vi "Chart[Template].TestLauncher.vi"() -> ()   [LabVIEW 2013, in "Chart[Template].lvclass"]
doc: "JKI State Machine Objects (SMO) 1.0.0.5\nJKI - JKI\nCopyright (c) 2016, JKI"
uses:
  Chart[Template].lvclass
  Typedefs/Dependencies--Cluster.ctl
  <vilib>/JKI/JKI SMO/SMO/SMO.lvclass
  <vilib>/JKI/JKI SMO/SMO.UI/SMO.UI.lvclass
panel:
  in  "Send":bool
  out "error out":errorcluster
  in  "Stop":bool
  # "Chart Test Launcher"
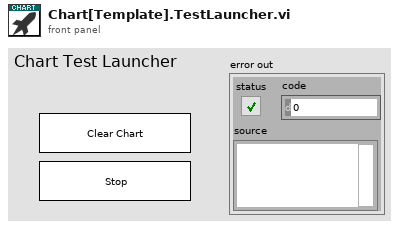
[diagram p1: front panel]
types:
  T1 = typedef "Chart[Template].lvclass/Dependencies--Cluster.ctl" = cluster{"SMO":refnum<class "SMO.lvclass">, "New Value":refnum<user-event>}
  T2 = cluster{"Chart[Template] Public Events":refnum<event-registration>, "SMO.UI Public Events":refnum<event-registration>}
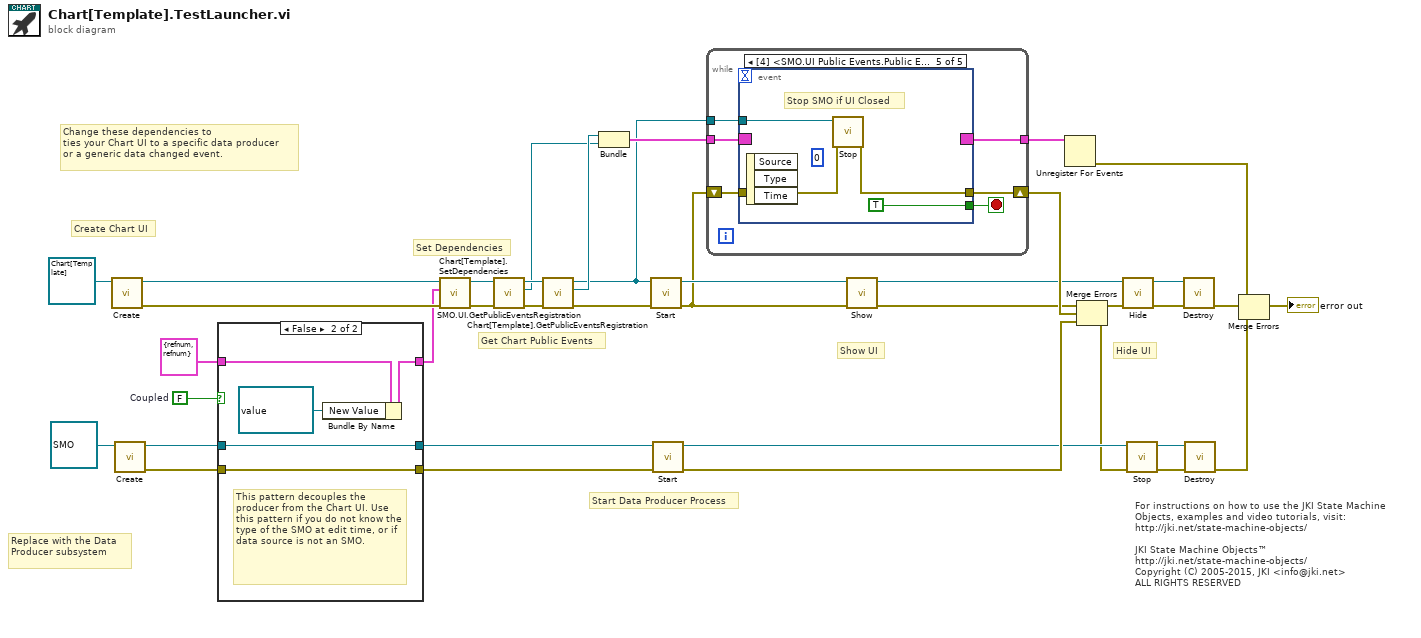
[diagram p0: block diagram]
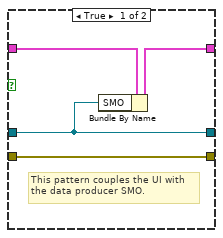
[diagram p2: hidden frame]
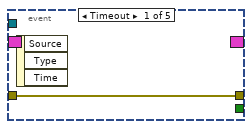
[diagram p3: hidden frame]
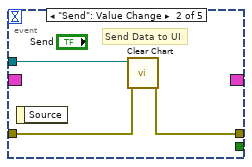
[diagram p4: hidden frame]
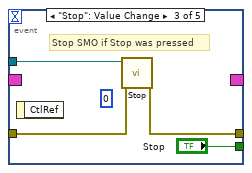
[diagram p5: hidden frame]
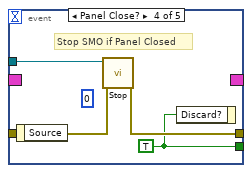
[diagram p6: hidden frame]
diagram:
  w5 = FALSE  # Coupled
  # "Start Data Producer Process"
  # "Set Dependencies"
  # "Create Chart UI"
  # "Replace with the Data Producer subsystem"
  # "Change these dependencies to\nties your Chart UI to a specific data producer\nor a generic data changed event."
  # "Hide UI"
  # "Show UI"
  # "For instructions on how to use the JKI State Machine Objects, examples and video tutorials, visit:\nhttp://jki.net/state-machine-objects/\n\nJKI State Machine Objects™\nhttp://jki.net/state-machine-objects/\nCopyright (C) 2005-2015, JKI <info@jki.net>\nALL RIGHTS RESERVED"
  # "Get Chart Public Events"
  n1 = call <vilib>:"Create.vi"("SMO"=refnum<class "Chart[Template].lvclass"> refnum ("Chart[Template]")) -> ("error out"=w16:errorcluster, "SMO out"=w18:refnum<class "Chart[Template].lvclass">)  [unwired: 8 in, 1 out]
  n2 = call <vilib>:"Create.vi"("SMO"=refnum<class "SMO.lvclass"> refnum) -> ("error out"=w1:errorcluster, "SMO out"=w4:refnum<class "SMO.lvclass">)  [unwired: 8 in, 1 out]
  n3 = case shown="False" w5 {
    tunnel: T1 {"SMO"=refnum, "New Value"=refnum} ("Dependencies") -> [w41 w46]
    tunnel: [w40 w45] -> w6
    tunnel: w4 -> [w39 w43]
    tunnel: [w39 w43] -> w3
    tunnel: [w38 w42] -> w2
    tunnel: w1 -> [w38 w42]
    frame True {
      # "This pattern couples the UI with\nthe data producer SMO."
      n4 = Bundle By Name(cluster=w41, "SMO"=w39) -> (w40:T1)
    }
    frame False {
      # "This pattern decouples the producer from the Chart UI. Use this pattern if you do not know the type of the SMO at edit time, or if data source is not an SMO."
      n5 = Bundle By Name(cluster=w46, "New Value"=refnum<user-event> refnum) -> (w45:T1)
    }
  }
  n6 = call "Chart[Template].SetDependencies.vi"("error in (no error)"=w16, "Dependencies"=w6, "Chart[Template]"=w18) -> ("error out"=w15:errorcluster, "Chart[Template] out"=w17:refnum<class "Chart[Template].lvclass">)  [unwired: 7 in]
  n7 = call <vilib>:"SMO.UI.GetPublicEventsRegistration.vi"("error in (no error)"=w15, "SMO.UI"=w17) -> ("error out"=w21:errorcluster, "SMO.UI Public Events"=w19:refnum<event-registration>, "SMO.UI out"=w20:refnum<class "Chart[Template].lvclass">)  [unwired: 7 in]
  n8 = call "Chart[Template].GetPublicEventsRegistration.vi"("error in (no error)"=w21, "Chart[Template]"=w20) -> ("error out"=w30:errorcluster, "Chart[Template] Public Events"=w29:refnum<event-registration>, "Chart[Template] out"=w28:refnum<class "Chart[Template].lvclass">)  [unwired: 7 in]
  n9 = Bundle("Chart[Template] Public Events"=w29, "SMO.UI Public Events"=w19) -> (w36:T2)  [unwired: 1 in]
  n10 = call <vilib>:"Start.vi"("error in (no error)"=w30, "SMO"=w28) -> ("error out"=w26:errorcluster, "SMO out"=w27:refnum<class "Chart[Template].lvclass">)  [unwired: 8 in]
  n11 = call <vilib>:"Start.vi"("error in (no error)"=w2, "SMO"=w3) -> ("error out"=w13:errorcluster, "SMO out"=w12:refnum<class "SMO.lvclass">)  [unwired: 8 in]
  n12 = while {
    shift-right: [w51] -> w35
    shift-left: w26 -> [w50]
    tunnel: w36 -> [w49]
    tunnel: [w48] -> w37
    tunnel: w28 -> [w47]
    stop <- w52 stop-if-true
    n13 = event shown="[4] <SMO.UI Public Events.Public Events.UI Hidden>: User Event" {
      selector: w49 -> [_ _ _ _ _]
      dyn-events: [_ _ _ _ _] -> w48
      timeout: _ -> [_ _ _ _ _]
      tunnel: [_ _ "Stop" w61 TRUE ("OK")] -> w52
      tunnel: w47 -> [_ w56 w58 w64 w68]
      tunnel: [w53 w54 w59 w63 w67] -> w51
      tunnel: w50 -> [w53 w55 w57 w62 w66]
      event Timeout {
        n14 = event-data() -> ()  [unwired: 1 in, 3 out]
      }
      event "Send": Value Change {
        # "Send Data to UI"
        n15 = event-data() -> ()  [unwired: 1 in, 1 out]
        n16 = call "Clear Chart.vi"("error in (no error)"=w55, "Chart[Template]"=w56) -> ("error out"=w54:errorcluster)  [unwired: 8 in, 1 out]
      }
      event "Stop": Value Change {
        (unwired) 0 ("timeout in ms (-1)")
        # "Stop SMO if Stop was pressed"
        n17 = event-data() -> ()  [unwired: 1 in, 1 out]
        n18 = call <vilib>:"Stop.vi"("error in (no error)"=w57, "SMO"=w58) -> ("error out"=w59:errorcluster)  [unwired: 8 in, 1 out]
      }
      event Panel Close? {
        (unwired) 0 ("timeout in ms (-1)")
        w61 = TRUE ("OK")
        # "Stop SMO if Panel Closed"
        n19 = event-data() -> ()  [unwired: 1 in, 1 out]
        n20 = call <vilib>:"Stop.vi"("error in (no error)"=w62, "SMO"=w64) -> ("error out"=w63:errorcluster)  [unwired: 8 in, 1 out]
        n21 = event-data("Discard?"=w61) -> ()  [unwired: 1 in, 1 out]
      }
      event User Event {
        (unwired) 0 ("timeout in ms (-1)")
        # "Stop SMO if UI Closed"
        n22 = event-data() -> ()  [unwired: 1 in, 3 out]
        n23 = call <vilib>:"Stop.vi"("error in (no error)"=w66, "SMO"=w68) -> ("error out"=w67:errorcluster)  [unwired: 8 in, 1 out]
      }
    }
  }
  n24 = call <vilib>:"Show.vi"("error in (no error)"=w26, "SMO.UI"=w27) -> ("error out"=w25:errorcluster, "SMO.UI out"=w24:refnum<class "Chart[Template].lvclass">)  [unwired: 8 in]
  n25 = Unregister For Events(event registration refnum=w37) -> (error out=w34:errorcluster)  [unwired: 1 in]
  n26 = Merge Errors(w25, w35, w13) -> (w11:errorcluster)
  n27 = call <vilib>:"Hide.vi"("error in (no error)"=w11, "SMO.UI"=w24) -> ("error out"=w22:errorcluster, "SMO.UI out"=w23:refnum<class "Chart[Template].lvclass">)  [unwired: 8 in]
  n28 = call <vilib>:"Stop.vi"("error in (no error)"=w11, "SMO"=w12) -> ("error out"=w10:errorcluster, "SMO out"=w9:refnum<class "SMO.lvclass">)  [unwired: 8 in]
  n29 = call <vilib>:"Destroy.vi"("error in (no error)"=w22, "SMO"=w23) -> ("error out"=w32:errorcluster)  [unwired: 9 in]
  n30 = call <vilib>:"Destroy.vi"("error in (no error)"=w10, "SMO"=w9) -> ("error out"=w8:errorcluster)  [unwired: 9 in]
  n31 = Merge Errors(w34, w32, w8) -> (→"error out":errorcluster)
